vi "Write Interlock message.vi"(8 "error in (no error)":errorcluster, 10 "Interlock message":string="Interlock!", 11 "Interlock in":refnum<class "Interlock.lvclass">) -> (0 "error out":errorcluster, 3 "Interlock out":refnum<class "Interlock.lvclass">)   [LabVIEW 2015, in "Interlocks.lvlib" / "Interlock.lvclass"]
uses:
  Interlock.lvclass
  Interlock.lvclass/Interlock.ctl
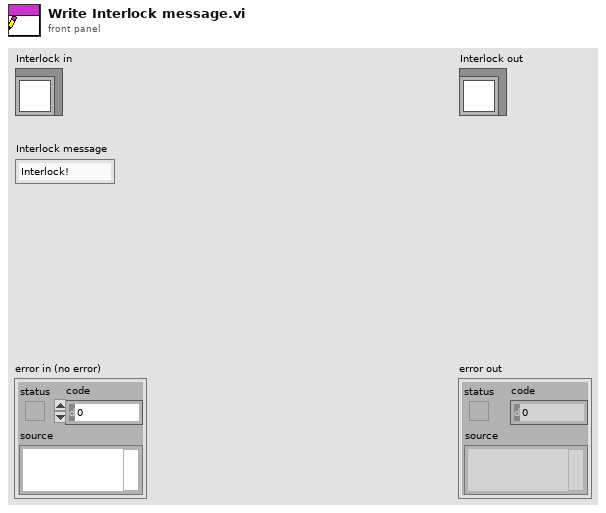
[diagram p1: front panel]
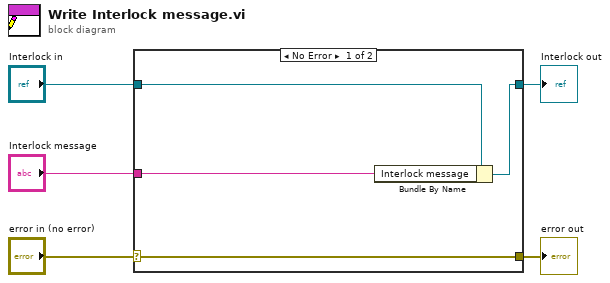
[diagram p0: block diagram]
diagram:
  n1 = case shown="No Error" "error in (no error)" {
    selector: "error in (no error)" -> [w9 w10]
    tunnel: [w9 w10] -> w4
    tunnel: [w7 w11] -> w2
    tunnel: "Interlock in" -> [w8 w11]
    tunnel: "Interlock message" -> [w6 _]
    frame No Error {
      n2 = Bundle By Name(cluster=w8, "Interlock message"=w6) -> (w7:refnum<class "Interlock.lvclass">)
    }
    frame Error {
    }
  }
  "error out" <- w4
  "Interlock out" <- w2
